vi "Init.vi"(8 "error in":errorcluster, 11 "TE Cooler in":refnum<class "TE Cooler.lvclass">) -> (0 "error out":errorcluster={"status"=TRUE, "code"=-1073807339, "source"="VISA Read in Serial IO.lvclass:Cmd to R_W - Synchronous.vi->TE Cooler.lvlib:TE Cooler.lvclass:Write to Port.vi->TE Cooler.lvlib:TE Cooler.lvclass:Init.vi->cPAS.lvclass:Serial Config.vi->cPAS.lvclass:Start Config.vi->PAS.lvclass:Configure.vi->PAS Server.vi->Combined Server.vi"}, 2 "SP":dbl, 3 "TE Cooler out":refnum<class "TE Cooler.lvclass">)   [LabVIEW 2015, in "TE Cooler.lvlib" / "TE Cooler.lvclass"]
doc: "Initialize the TE Cooler using the parameters already entered for PID control and heater power."
uses:
  TE Cooler.lvclass
  Controls/Command.ctl
  Configurable Device/Configurable Device.lvclass/Configurable Device.ctl
  reusable/Session APIs/File Access/Config Data/Config Data.lvclass/Config Data.ctl
  Configurable Device/Read Handle.vi
  reusable/Session APIs/File Access/Config Data/Accessors/Read Ref.vi
  Configurable Device/Accessors/Write Addr.vi
  <vilib>/Utility/config.llb/Read Key (String).vi
  <vilib>/Utility/config.llb/Read Key (Double).vi
  reusable/Session APIs/File Access/Config Data/Config Data.lvclass
  <vilib>/Utility/config.llb/NI_LVConfig.lvlib
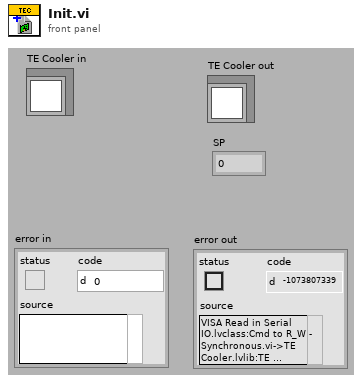
[diagram p1: front panel]
types:
  T1 = typedef "TE Cooler.lvlib/TE Cooler.lvclass/Command.ctl" = enum16{"INPUT1", "DESIRED CONTROL VALUE", "POWER OUTPUT", "ALARM STATUS", "INPUT 2", "OUTPUT CURRENT COUNTS", "ALARM TYPE", "SET TYPE DEFINE", "SENSOR TYPE", "CONTROL TYPE", "CONTROL OUTPUT POLARITY", "POWER ON/OFF", "OUTPUT SHUTDOWN IF ALARM", "FIXED DESIRED CONTROL SETTING", "PROPORTIONAL BANDWIDTH", "INTEGRAL GAIN", "DERIVATIVE GAIN", "LOW EXTERNAL SET RANGE", "HIGH EXTERNAL SET RANGE", "ALARM DEADBAND", "HIGH ALARM SETTING", "LOW ALARM SETTING", "CONTROL DEADBAND SETTING", "INPUT1 OFFSET", "INPUT2 OFFSET", "HEAT MULTIPLIER", "COOL MULTIPLIER", "OVER CURRENT COUNT COMPARE VALUE", "ALARM LATCH ENABLE", "NOT USED", "ALARM LATCH RESET", "CHOOSE SENSOR FOR ALARM FUNCTION", "CHOOSE TEMPERATURE WORKING UNITS", "EEPROM WRITE ENABLE", "OVER CURRENT CONTINUOUS", "OVER CURRENT RESTART ATTEMPTS", "JP3 DISPLAY ENABLE"}
  T2 = typedef "Config Data.lvclass/Config Session.ctl" = refnum<data-value>
  T3 = typedef "NI_LVConfig.lvlib/Config Data RefNum.ctl" = refnum<k1>
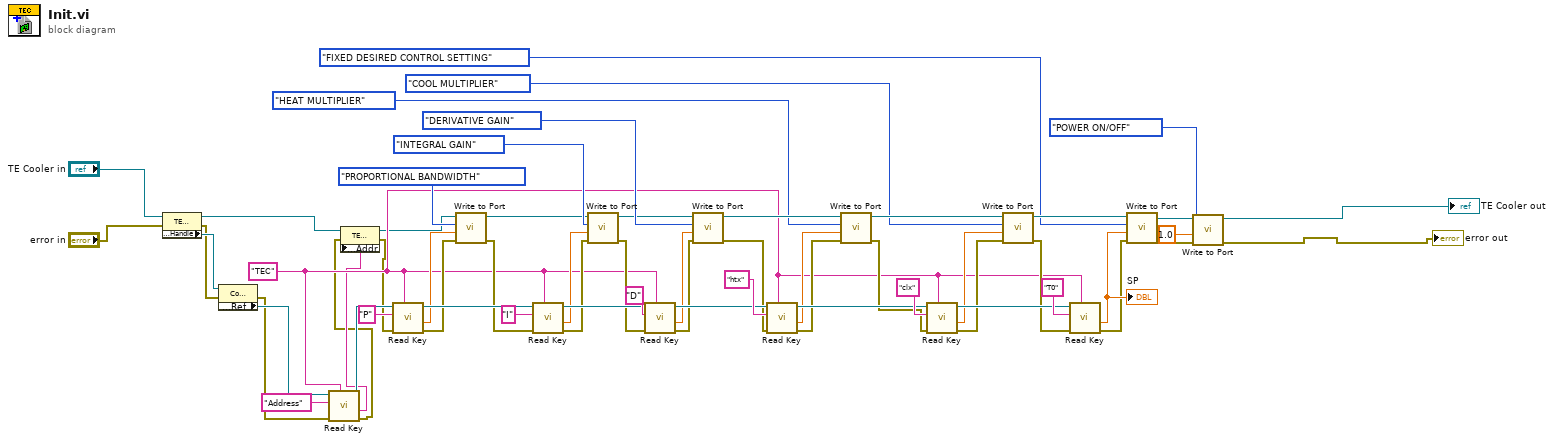
[diagram p0: block diagram]
diagram:
  w12 = "TEC" ("section")
  n1 = property class="TE Tech"(reference="TE Cooler in", error in="error in") -> (reference out=w11:refnum<class "TE Cooler.lvclass">, error out=w45:errorcluster, "Accessors:Handle"=w47:T2)
  n2 = property class="Config Data"(reference=w47, error in=w45) -> (error out=w14:errorcluster, "Accessors:Ref"=w16:T3)  [unwired: 1 out]
  n3 = call-poly <vilib>:"Read Key.vi"("section"=w12, "error in (no error)"=w14, "key"="Address", "refnum"=w16) -> ("error out"=w8:errorcluster, "value"=w9:string, "refnum out"=w15:T3)  [unwired: 4 in, 1 out]
  n4 = property class="TE Tech"(reference=w11, error in=w8, "Accessors:Addr"=w9) -> (reference out=w10:refnum<class "TE Cooler.lvclass">, error out=w7:errorcluster)
  n5 = call-poly <vilib>:"Read Key.vi"("section"=w12, "error in (no error)"=w7, "key"="P", "refnum"=w15) -> ("error out"=w27:errorcluster, "value"=w34:dbl, "refnum out"=w42:T3)  [unwired: 4 in, 1 out]
  n6 = call "Write to Port.vi"("error in"=w27, "Input Value"=w34, "TEC Cmd"=Command."PROPORTIONAL BANDWIDTH", "TE Cooler in"=w10) -> ("error out"=w26:errorcluster, "TE Cooler out"=w56:refnum<class "TE Cooler.lvclass">)  [unwired: 5 in, 1 out]
  n7 = call-poly <vilib>:"Read Key.vi"("section"=w12, "error in (no error)"=w26, "key"="I", "refnum"=w42) -> ("error out"=w25:errorcluster, "value"=w33:dbl, "refnum out"=w41:T3)  [unwired: 4 in, 1 out]
  n8 = call "Write to Port.vi"("error in"=w25, "Input Value"=w33, "TEC Cmd"=Command."INTEGRAL GAIN", "TE Cooler in"=w56) -> ("error out"=w24:errorcluster, "TE Cooler out"=w55:refnum<class "TE Cooler.lvclass">)  [unwired: 5 in, 1 out]
  n9 = call-poly <vilib>:"Read Key.vi"("section"=w12, "error in (no error)"=w24, "key"="D", "refnum"=w41) -> ("error out"=w22:errorcluster, "value"=w32:dbl, "refnum out"=w37:T3)  [unwired: 4 in, 1 out]
  n10 = call "Write to Port.vi"("error in"=w22, "Input Value"=w32, "TEC Cmd"=Command."DERIVATIVE GAIN", "TE Cooler in"=w55) -> ("error out"=w23:errorcluster, "TE Cooler out"=w54:refnum<class "TE Cooler.lvclass">)  [unwired: 5 in, 1 out]
  n11 = call-poly <vilib>:"Read Key.vi"("section"=w12, "error in (no error)"=w23, "key"="htx", "refnum"=w37) -> ("error out"=w21:errorcluster, "value"=w31:dbl, "refnum out"=w36:T3)  [unwired: 4 in, 1 out]
  n12 = call "Write to Port.vi"("error in"=w21, "Input Value"=w31, "TEC Cmd"=Command."HEAT MULTIPLIER", "TE Cooler in"=w54) -> ("error out"=w20:errorcluster, "TE Cooler out"=w53:refnum<class "TE Cooler.lvclass">)  [unwired: 5 in, 1 out]
  n13 = call-poly <vilib>:"Read Key.vi"("section"=w12, "error in (no error)"=w20, "key"="clx", "refnum"=w36) -> ("error out"=w19:errorcluster, "value"=w30:dbl, "refnum out"=w35:T3)  [unwired: 4 in, 1 out]
  n14 = call "Write to Port.vi"("error in"=w19, "Input Value"=w30, "TEC Cmd"=Command."COOL MULTIPLIER", "TE Cooler in"=w53) -> ("error out"=w18:errorcluster, "TE Cooler out"=w50:refnum<class "TE Cooler.lvclass">)  [unwired: 5 in, 1 out]
  n15 = call-poly <vilib>:"Read Key.vi"("section"=w12, "error in (no error)"=w18, "key"="T0", "refnum"=w35) -> ("error out"=w17:errorcluster, "value"=w29:dbl)  [unwired: 4 in, 2 out]
  "SP" <- w29
  n16 = call "Write to Port.vi"("error in"=w17, "Input Value"=w29, "TEC Cmd"=Command."FIXED DESIRED CONTROL SETTING", "TE Cooler in"=w50) -> ("error out"=w5:errorcluster, "TE Cooler out"=w6:refnum<class "TE Cooler.lvclass">)  [unwired: 5 in, 1 out]
  n17 = call "Write to Port.vi"("error in"=w5, "Input Value"=1.0, "TEC Cmd"=Command."POWER ON/OFF", "TE Cooler in"=w6) -> ("error out"=→"error out":errorcluster, "TE Cooler out"=→"TE Cooler out":refnum<class "TE Cooler.lvclass">)  [unwired: 5 in, 1 out]
